vi "Connect Newport Instruments_libESP301.vi"(4 "XON/XOFF (False)":bool, 6 "Baud Rate (921600 - USB)":u32=921600 min=300 max=115200 step=300, 7 "Filter Term for Instruments (\"\" - none)":string, 8 "error in (no error)":errorcluster) -> (0 "error (duplicate)":errorcluster, 1 "Connected":bool, 2 "VISA resource name (duplicate)":refnum<visa-resource-name>, 3 "Device Connection Cluster":T1, 5 "GPIB? ( T - GPIB, F - RS232 )":bool)   [LabVIEW 2012, in "Newport ESP301.lvlib"]
doc: "Connect Newport Device\n\nGet list of instrument, filter (if set) and allow for selection of device to talk to.\n\nThis is generic selection of the instrument to connected to, so look in system settings or on device to verify it is the correct port."
uses:
  Newport ESP301.lvlib
panel:
  # "s"
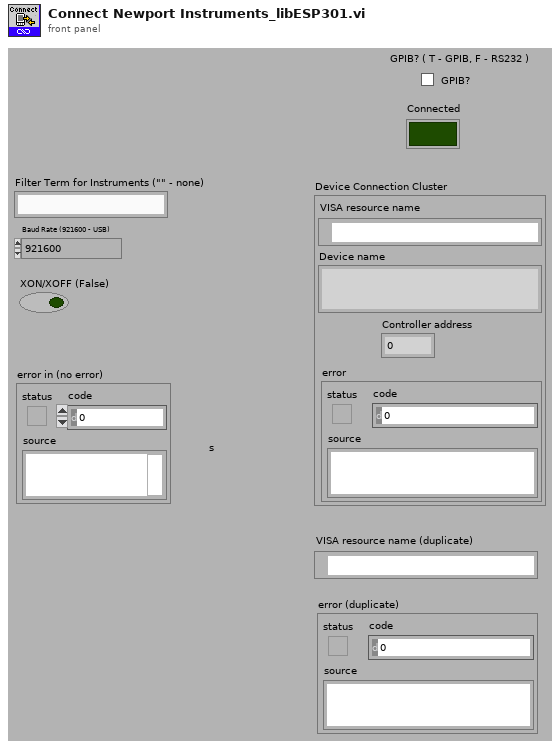
[diagram p1: front panel]
types:
  T1 = cluster{"VISA resource name":refnum<visa-resource-name>, "Device name":string, "Controller address":i32, "error":errorcluster}
  T2 = cluster{"VISA resource name":refnum<visa-resource-name>, "result string":string, "Controller address":i32, "error out":errorcluster}
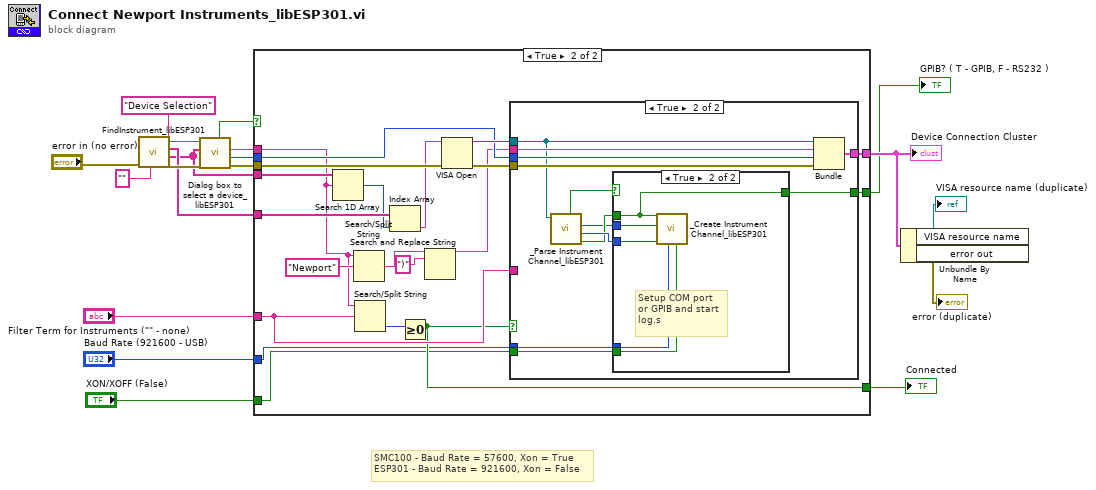
[diagram p0: block diagram]
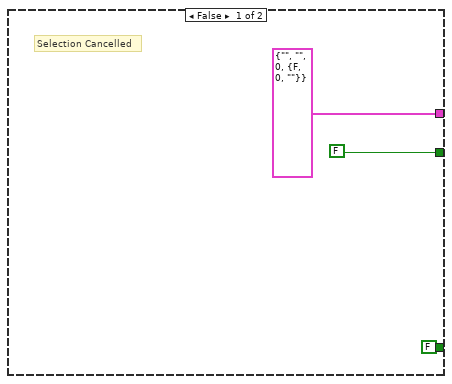
[diagram p2: hidden frame]
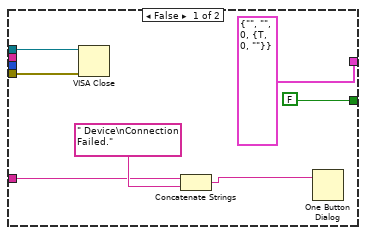
[diagram p3: hidden frame]
diagram:
  # "SMC100 - Baud Rate = 57600, Xon = True\nESP301 - Baud Rate = 921600, Xon = False"
  n1 = call "FindInstrument_libESP301.vi"("search string/char ()"="" ("search string/char (-)"), "error in (no error)"="error in (no error)") -> ("error out"=w17:errorcluster, "Found Interface Names"=w14:string[], "Found Resource Names"=w16:string[])  [unwired: 7 in]
  n2 = call "Dialog box to select a device_libESP301.vi"("Error IN"=w17, "Connected devices"=w14, "Title"="Device Selection") -> ("Error OUT"=w15:errorcluster, "Controller address"=w13:i32, "Selected device"=w12:string, "OK?"=w11:bool)  [unwired: 3 in]
  n3 = case shown="True" w11 {
    tunnel: w16 -> [_ w41]
    tunnel: w15 -> [_ w40]
    tunnel: w14 -> [_ w39]
    tunnel: w13 -> [_ w35]
    tunnel: [T2 {"VISA resource name"="", "result string"="", "Controller address"=0, "error out"={"status"=FALSE, "code"=0, "source"=""}} w33] -> w4
    tunnel: w12 -> [_ w28]
    tunnel: "Filter Term for Instruments (\"\" - none)" -> [_ w26]
    tunnel: [FALSE w25] -> w9
    tunnel: "Baud Rate (921600 - USB)" -> [_ w24]
    tunnel: "XON/XOFF (False)" -> [_ w23]
    tunnel: [FALSE w22] -> w1
    frame False {
      # "Selection Cancelled"
    }
    frame True {
      n4 = Search 1D Array(1D array=w39, element=w28) -> (index of element=w38:i32)  [unwired: 1 in]
      n5 = Search/Split String(string=w28, search string/char (-)="Newport") -> (match + rest of string=w31:string)  [unwired: 1 in, 2 out]
      n6 = Search/Split String(string=w28, search string/char (-)=w26) -> (offset of match=w27:i32)  [unwired: 1 in, 2 out]
      n7 = Index Array(array=w41, index=w38) -> (element=w36:string)
      n8 = Greater Or Equal To 0?(x=w27) -> (x >= 0?=w25:bool)
      n9 = Search and Replace String(input string=w31, search string=")") -> (result string=w29:string)  [unwired: 6 in, 3 out]
      n10 = VISA Open(error in (no error)=w40, VISA resource name=w36) -> (VISA resource name=w37:refnum<visa-resource-name>, error out=w34:errorcluster)  [unwired: 3 in]
      n11 = case shown="True" w25 {
        tunnel: w37 -> [w47 w56]
        tunnel: w35 -> [_ w60]
        tunnel: w34 -> [w46 w59]
        tunnel: [T2 {"VISA resource name"="", "result string"="", "Controller address"=0, "error out"={"status"=TRUE, "code"=0, "source"=""}} w58] -> w33
        tunnel: w29 -> [_ w57]
        tunnel: w26 -> [w43 _]
        tunnel: w24 -> [_ w52]
        tunnel: w23 -> [_ w49]
        tunnel: [FALSE w50] -> w22
        frame False {
          n12 = VISA Close(VISA resource name=w47, error in (no error)=w46) -> ()  [unwired: 1 out]
          n13 = Concatenate Strings(w43, " Device\nConnection Failed." ("message")) -> (w45:string)
          n14 = One Button Dialog(message=w45) -> ()  [unwired: 1 in, 1 out]
        }
        frame True {
          n15 = call "_Parse Instrument Channel_libESP301.vi"("Instrument Channel"=w56) -> ("T - GPIB, F - RS232"=w54:bool, "Hardware Address"=w55:i32, "Instrument Address"=w53:i16, "Valid String"=w51:bool)  [unwired: 6 in, 1 out]
          n16 = case shown="True" w51 {
            selector: w51 -> [w61 _]
            tunnel: w55 -> [_ w66]
            tunnel: w54 -> [_ w63]
            tunnel: w53 -> [_ w65]
            tunnel: w52 -> [_ w64]
            tunnel: [w61 w63] -> w50
            tunnel: w49 -> [_ w62]
            frame False {
            }
            frame True {
              # "Setup COM port\nor GPIB and start\nlog.s"
              n17 = call "_Create Instrument Channel_libESP301.vi"("XON/XOFF (False)"=w62, "Baud Rate (921600 - USB)"=w64, "COM Port (1)"=w66, "GPIB Primary Address (4)"=w65, "(F), T - GPIB, F - RS232"=w63) -> ()  [unwired: 4 in, 3 out]
            }
          }
          n18 = Bundle("VISA resource name"=w56, "result string"=w57, "Controller address"=w60, "error out"=w59) -> (w58:T2)  [unwired: 1 in]
        }
      }
    }
  }
  "Device Connection Cluster" <- w4
  "Connected" <- w9
  "GPIB? ( T - GPIB, F - RS232 )" <- w1
  n19 = Unbundle By Name(w4) -> ("VISA resource name"=→"VISA resource name (duplicate)":refnum<visa-resource-name>, "error out"=→"error (duplicate)":errorcluster)
